vi "Pulse Accq -unphuck.vi"() -> ()   [LabVIEW 2009]
uses:
  5122-States.ctl
  <vilib>/Utility/file.llb/Write To Spreadsheet File (DBL).vi
  <instrlib>/niScope/Configure/Trigger/niScope Configure Trigger Edge.vi
  <instrlib>/niScope/Acquire/Fetch/niScope Multi Fetch WDT.vi
  <instrlib>/niScope/Controls/niScope vertical coupling.ctl
panel:
  out "wfm info":T1(array[cluster]) {"reserved2" format="%.2f"; "reserved1" format="%.2f"; "offset" format="%^.3e"; "gain" format="%^.3e"; "xIncrement" format="%^.3e"; "relativeInitialX" format="%^.3e"; "absoluteInitialX" format="%^.3e"}
  out "# Acquired":i32=100 caption="Number of Records Acquired"
  out "# Fetched":i32=100 caption="Number of Records Fetched"
  out "Last Record Fetched":waveform(dbl)[](graph)
  in  "Plot Data?":bool=TRUE
  out "error out":errorcluster {"code" format="%.0x"}
  out "sample mode":i32
  out "Acquisition Sequence":dbl[][](graph)
  out "Total Acquired Time":dbl[unit]
  out "Total Number of Datapoints":i32=1000000
  out "Total Experiment Time":dbl[unit]
  in  "Number of Pulses to Record":i32=1 caption="Number of Runs" format="%.0p"
  out "Raman Measurement File Root":path
  out "Phase-Frequency Pairs":path
  out "Shot Noise File":path
  out "Reference Pulse File":path
  out "Quadrature Pulses File":path
  out "Raw Phase, Trigger, Extracted Phase Data":path
  out "Data Directory":path
  out "Writing Phase to File":bool
  in  "Master Stop":bool
  in  "Memory Repetition Period":dbl[unit]=0.025
  out "Actual Sample Rate":dbl[unit]
  in  "Get Reference Parameters":bool
  out "Reference Pulse":dbl[](array[numeric])
  in  "Capture":bool
  out "Acquisitions Remaining":i32 caption="Number of Runs"
  out "Number of Samples per Pulse":i32
  in  "Vertical range (0 to 10V)":dbl[unit]=4.0 caption="Vertical Range (V)" format="%.2f"
  in  "Desired Sample Rate":dbl[unit]=100000000.0 caption="Min. Sample Rate" step=1.0 format="%.2p"
  in  "Vertical coupling":T2=1 caption="Vertical Coupling" items=["AC", "DC", "Ground"]
  in  "Acquisition Delay":dbl[unit] format="%.2f"
  in  "Channel":u16(ring) items=["0", "1"]
  out "Channel String":string
  in  "Acquisition Time per Pulse":dbl[unit]=0.0005 format="%#.2g"
  in  "Acquire Data":bool
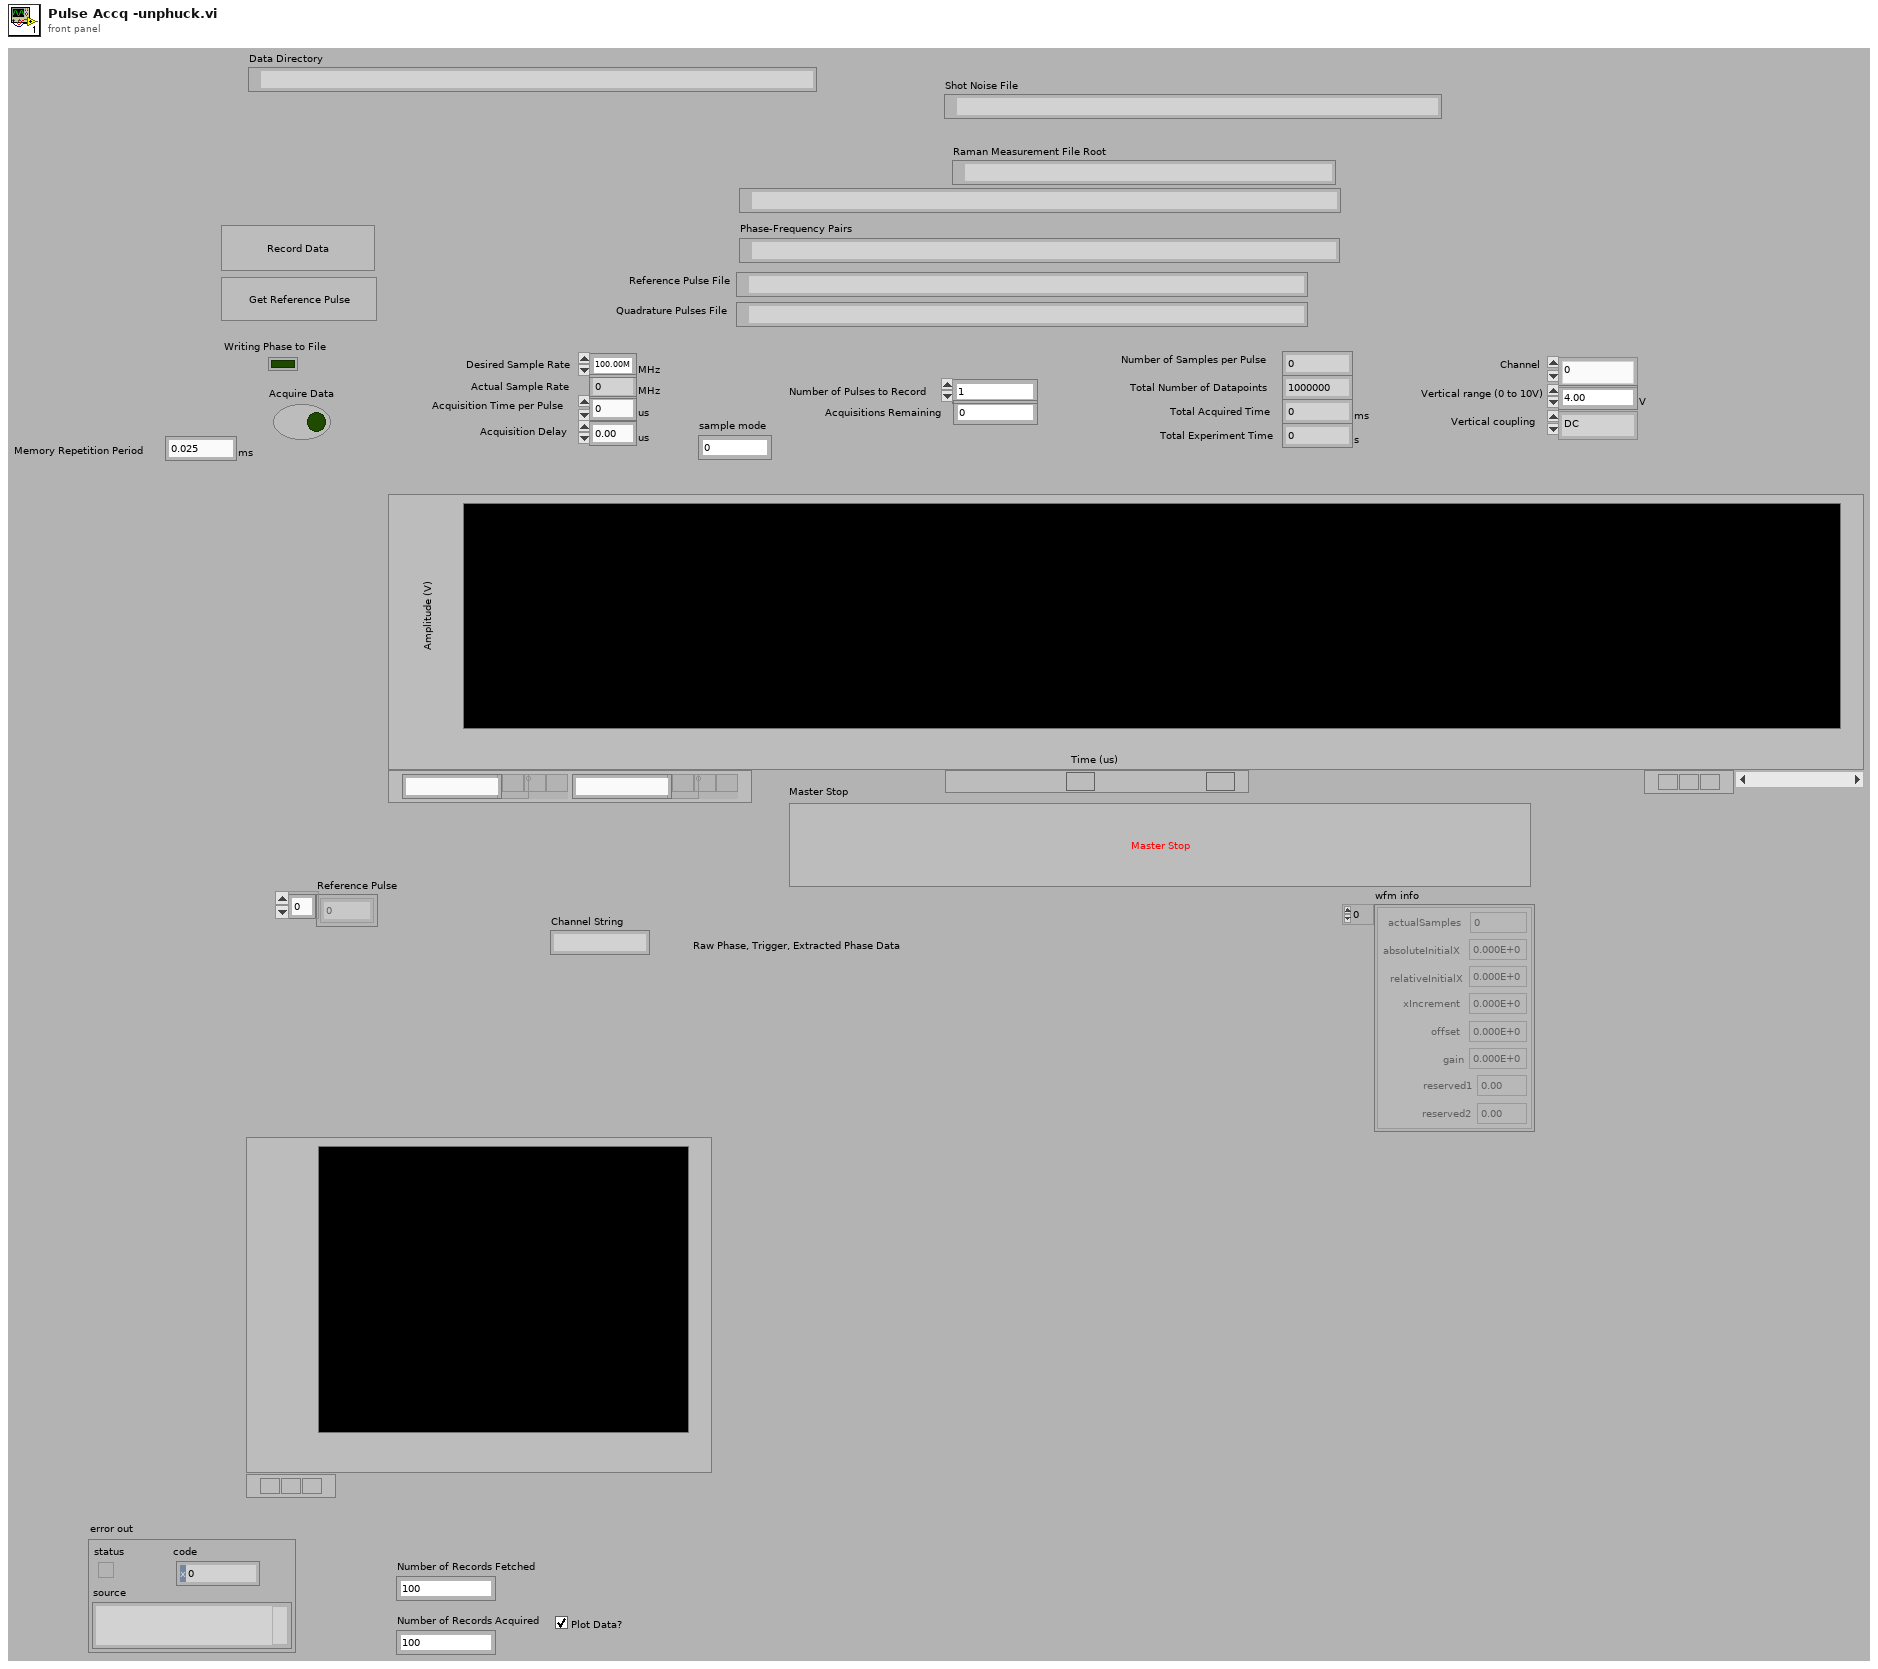
[diagram p1: front panel]
types:
  T1 = cluster{"actualSamples":i32, "absoluteInitialX":dbl, "relativeInitialX":dbl, "xIncrement":dbl, "offset":dbl, "gain":dbl, "reserved1":dbl, "reserved2":dbl}[]
  T2 = typedef "niScope vertical coupling.ctl" = i32
  T3 = enum16{"open", "open or create", "create or replace", "create", "open (read-only)"}
  T4 = enum16{"open", "replace", "create", "open or create", "replace or create", "replace or create with confirmation"}
  T5 = typedef "5122-States.ctl" = enum16{"Initialize Card", "Continuous Mode", "Fetch", "Snapshot Acquistion", "Standby", "Record DataFile", "Exit"}
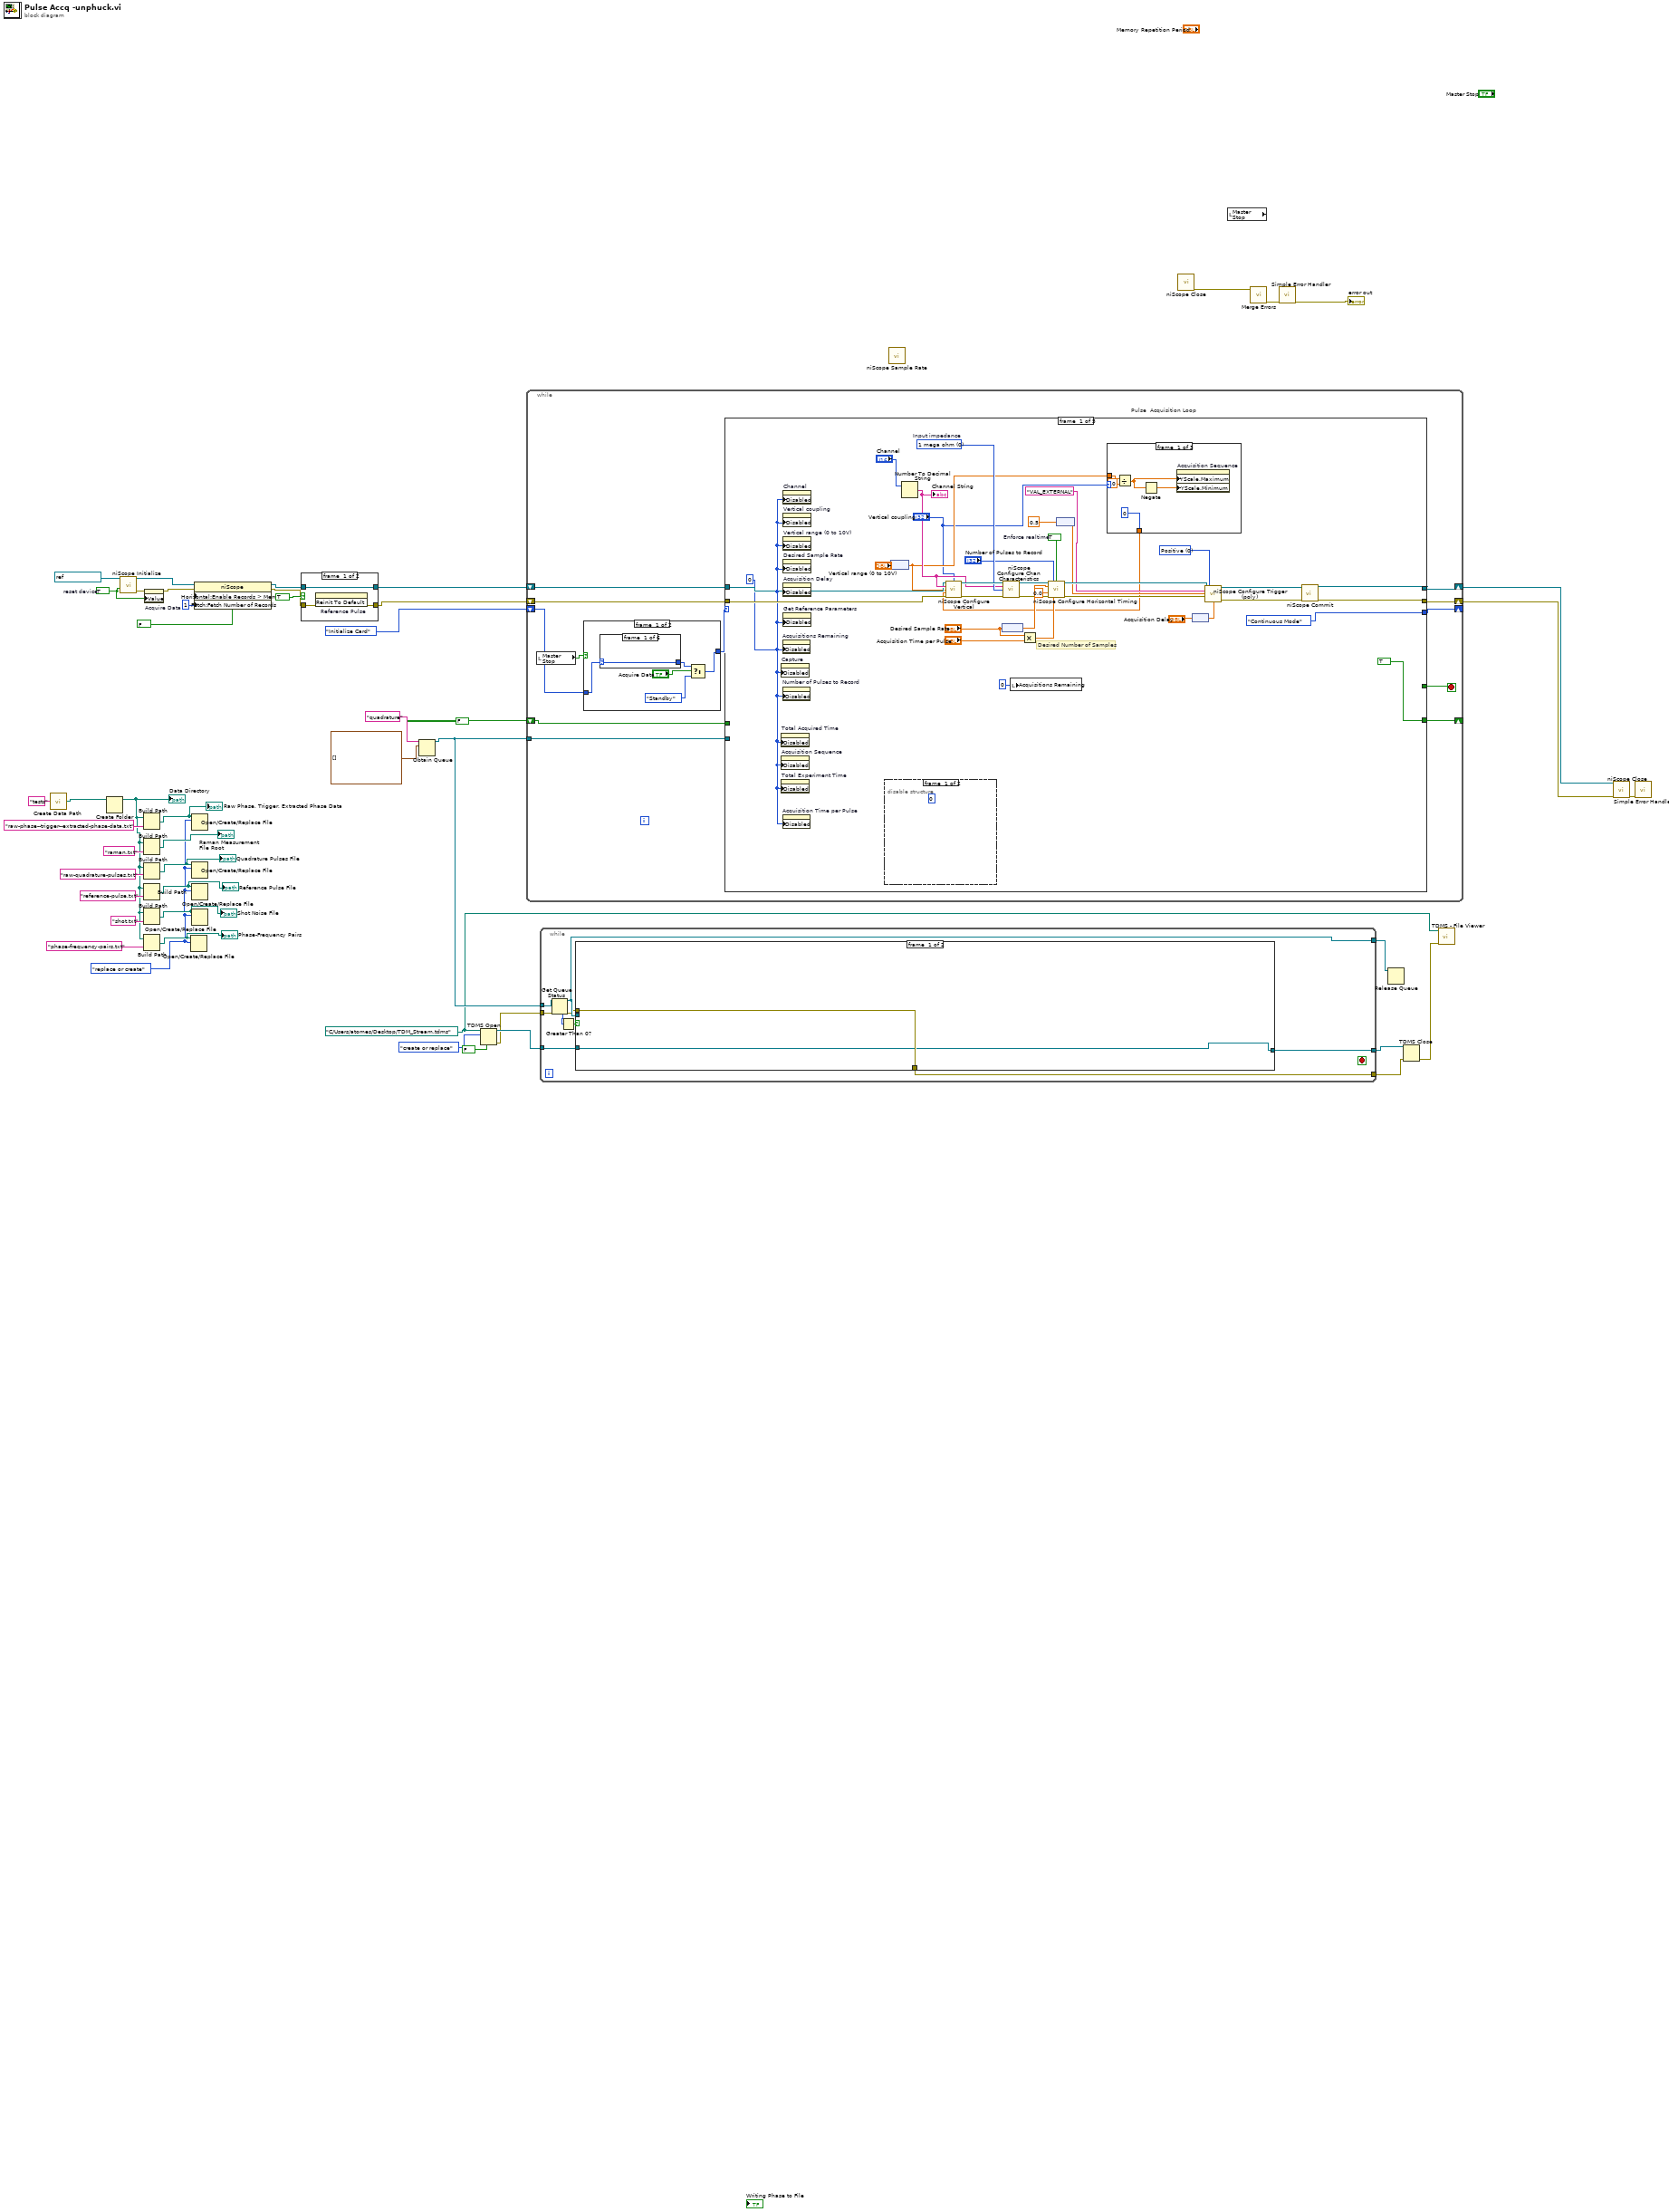
[diagram p0: block diagram]
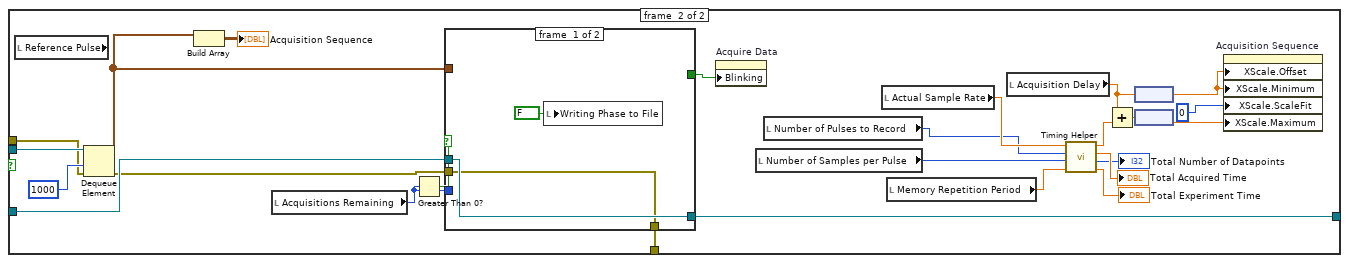
[diagram p2: hidden frame]
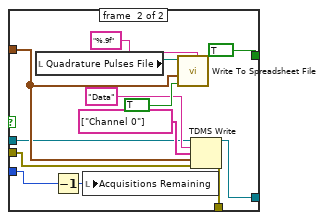
[diagram p3: hidden frame]
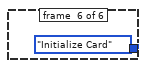
[diagram p9: hidden frame]
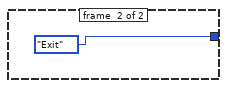
[diagram p10: hidden frame]
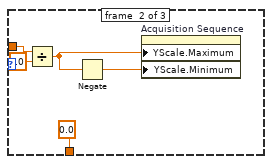
[diagram p12: hidden frame]
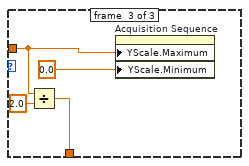
[diagram p13: hidden frame]
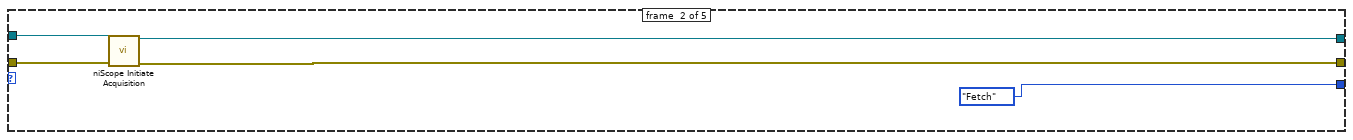
[diagram p14: hidden frame]
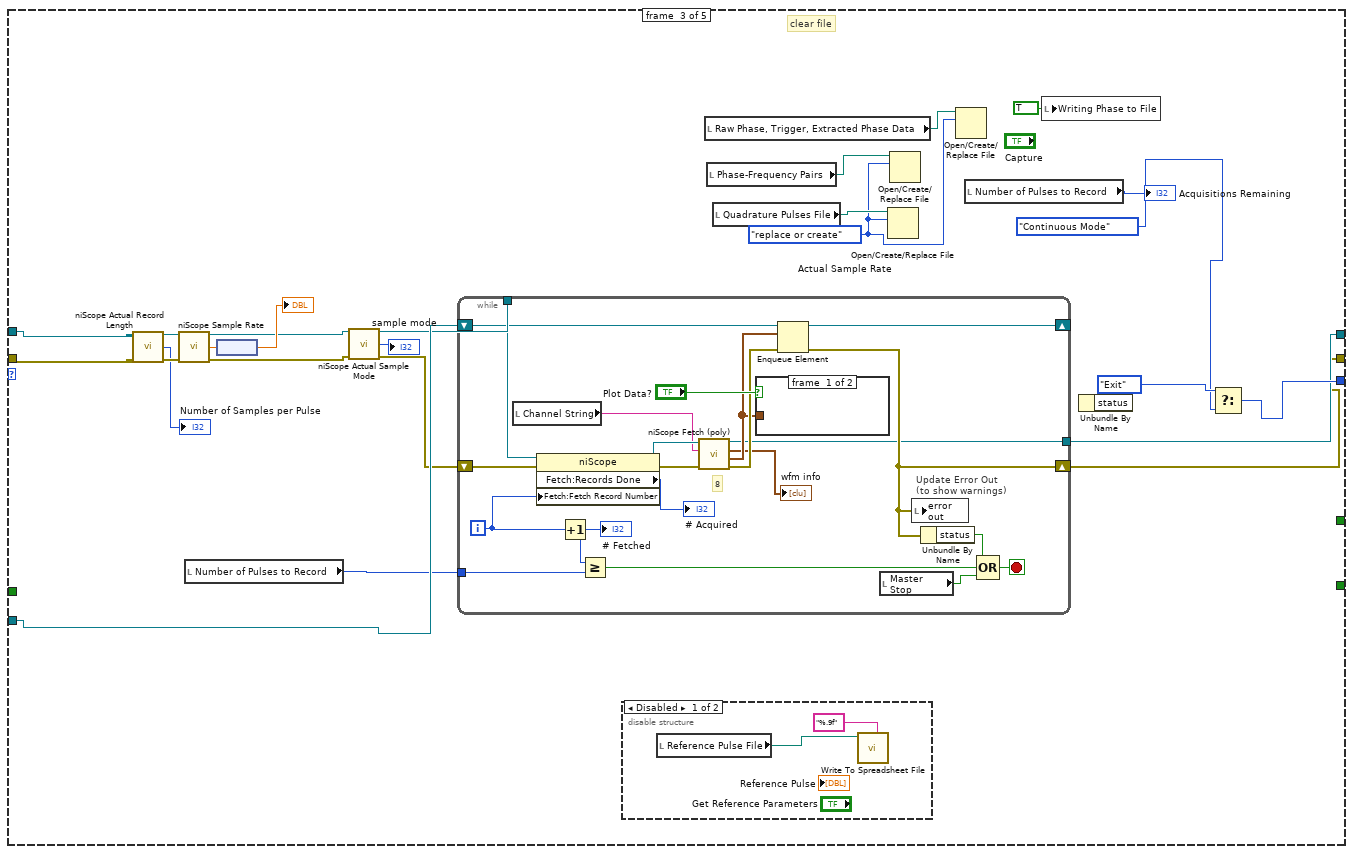
[diagram p15: hidden frame]
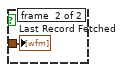
[diagram p17: hidden frame]
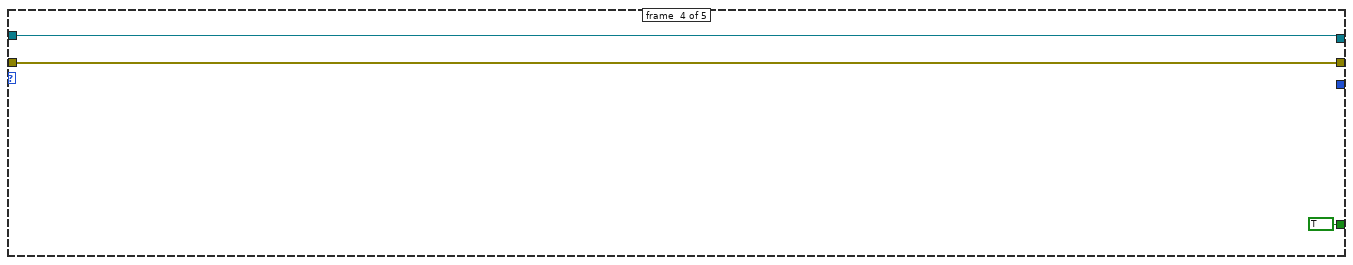
[diagram p18: hidden frame]
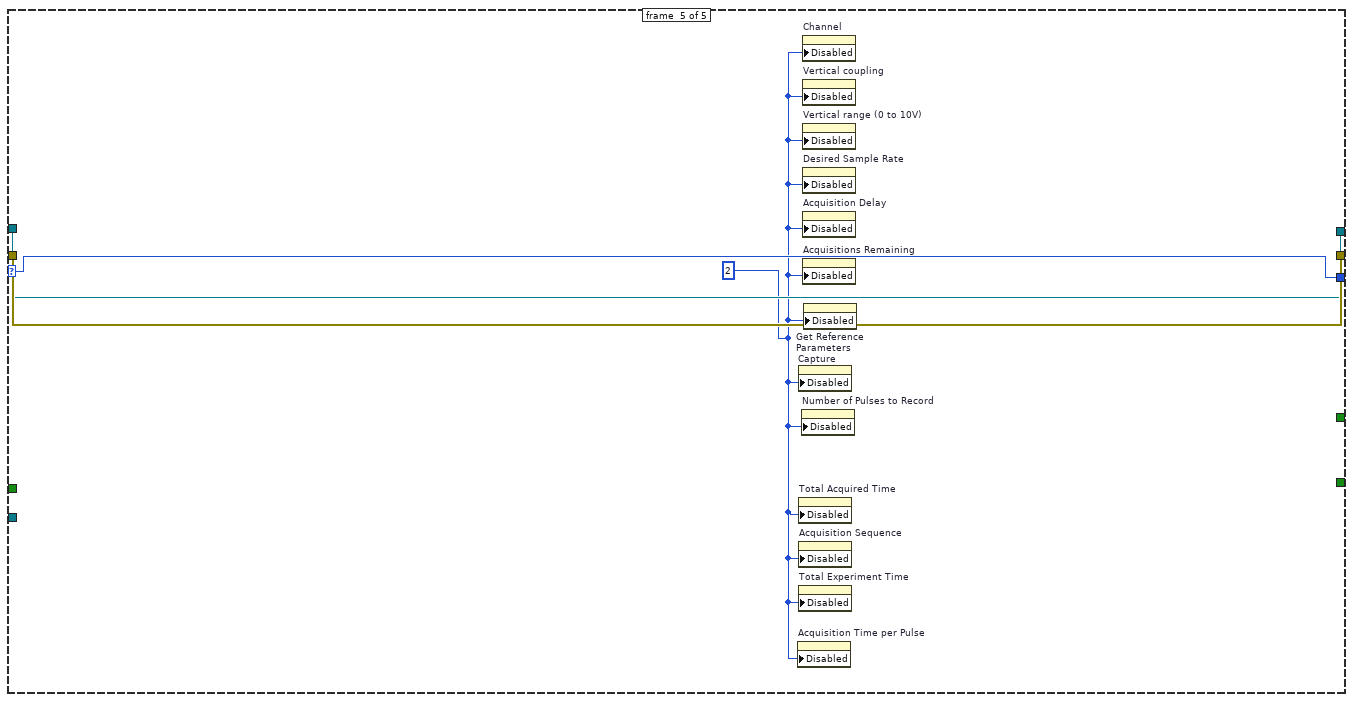
[diagram p19: hidden frame]
diagram:
  w4 = path "C:/Users/atomes/Desktop/TDM_Stream.tdms" ("selected path")
  w25 = T4."replace or create" ("operation (0:open)")
  w46 = TRUE  # reset device
  n1 = call "Create Data Path.vi"("Data Directory Name"="tests") -> ("appended path"=w36:path)
  n2 = Create Folder(path (use dialog)=w36) -> (created path=w27:path)  [unwired: 2 in, 2 out]
  "Data Directory" <- w27
  n3 = call <instrlib>:"niScope Initialize.vi"("resource name"=refnum<k15> "Acquisition" ("Resource name 5"), "reset device"=w46) -> ("instrument handle"=w17:refnum<k15>, "error out"=w47:errorcluster)  [unwired: 2 in, 10 out]
  n4 = Build Path(base path=w27, name or relative path="raw-phase--trigger--extracted-phase-data.txt") -> (appended path=w34:path)
  "Raw Phase, Trigger, Extracted Phase Data" <- w34
  n5 = Build Path(base path=w27, name or relative path="raman.txt") -> (appended path=→"Raman Measurement File Root":path)
  n6 = Build Path(base path=w27, name or relative path="raw-quadrature-pulses.txt") -> (appended path=w32:path)
  "Quadrature Pulses File" <- w32
  n7 = Build Path(base path=w27, name or relative path="reference-pulse.txt") -> (appended path=w31:path)
  "Reference Pulse File" <- w31
  n8 = Build Path(base path=w27, name or relative path="shot.txt") -> (appended path=w30:path)
  "Shot Noise File" <- w30
  n9 = Build Path(base path=w27, name or relative path="phase-frequency-pairs.txt") -> (appended path=w26:path)
  "Phase-Frequency Pairs" <- w26
  n10 = property on="Acquire Data" class="Bool (strict)"(error in=w47, "Value"=w46) -> (error out=w14:errorcluster)  [unwired: 1 in, 1 out]
  n11 = Open/Create/Replace File(file path (use dialog)=w26, operation (0:open)=w25) -> ()  [unwired: 4 in, 3 out]
  n12 = Open/Create/Replace File(file path (use dialog)=w34, operation (0:open)=w25) -> ()  [unwired: 4 in, 3 out]
  n13 = Open/Create/Replace File(file path (use dialog)=w32, operation (0:open)=w25) -> ()  [unwired: 4 in, 3 out]
  n14 = Open/Create/Replace File(file path (use dialog)=w31, operation (0:open)=w25) -> ()  [unwired: 4 in, 3 out]
  n15 = Open/Create/Replace File(file path (use dialog)=w30, operation (0:open)=w25) -> ()  [unwired: 4 in, 3 out]
  n16 = property class="niScope"(reference=w17, error in=w14, "Horizontal:Enable Records > Memory"=FALSE, "Fetch:Fetch Number of Records"=1) -> (reference out=w16:refnum<k15>, error out=w15:errorcluster)
  n17 = case shown="True" TRUE {
    tunnel: [w50 w52] -> w43
    tunnel: w16 -> [w50 w52]
    tunnel: [w49 w51] -> w42
    tunnel: w15 -> [w49 w51]
    frame #0 {
      n18 = invoke on="Reference Pulse" class="Arr (strict)" method="Reinit To Default"() -> ()  [unwired: 3 in, 3 out]
    }
    frame #1 {
    }
  }
  n19 = Obtain Queue(name (unnamed)="quadrature", element data type=waveform(dbl)[] [] ("wfm")) -> (queue out=w23:refnum<queue>)  [unwired: 3 in, 2 out]
  n20 = TDMS Open(6:FALSE ("disable buffering (T)"), 10:T3."create or replace" ("operation"), 11:w4) -> (0:w7:errorcluster, 3:w10:refnum<k34>)  [unwired: 3 in]
  n21 = while {
    shift-right: [w59] -> _
    shift-left: 5122-States."Initialize Card" ("Enum") -> [w57]
    shift-right: [w64] -> w21
    shift-left: w43 -> [w62]
    shift-right: [w63] -> w22
    shift-left: w42 -> [w61]
    shift-right: [w56] -> _
    shift-left: FALSE -> [w55]
    tunnel: w23 -> [w53]
    stop <- w60 stop-if-true
    # "Pulse  Acquisition Loop"
    n22 = local read "Master Stop"() -> (w54:bool)
    n23 = case shown="False" w54 {
      tunnel: [w66 5122-States."Exit" ("Enum")] -> w58
      tunnel: w57 -> [w69 _]
      frame #0 {
        n24 = case shown="\"Continuous Mode\"" w69 {
          selector: w69 -> [w70 w71 w72 w73 w74 _]
          tunnel: [w70 w71 w72 w73 w74 5122-States."Initialize Card" ("Enum")] -> w68
          frame #0 {
          }
          frame #1 {
          }
          frame #2 {
          }
          frame #3 {
          }
          frame #4 {
          }
          frame #5 {
          }
        }
        n25 = Select(t=w68, s="Acquire Data", f=5122-States."Standby" ("Enum")) -> (s? t:f=w66:T5)
      }
      frame #1 {
      }
    }
    n26 = case shown="\"Fetch\"" w58 {
      selector: w58 -> [_ _ _ _ w186]
      tunnel: [w94 w129 w140 w184 w187] -> w64
      tunnel: [w93 w130 w139 w183 w188] -> w63
      tunnel: w62 -> [w96 w132 w146 w184 w187]
      tunnel: w61 -> [w95 w131 w145 w183 w188]
      tunnel: [5122-States."Continuous Mode" ("Enum") 5122-States."Fetch" ("Enum") w157 _ w186] -> w59
      tunnel: [_ _ _ TRUE ("Acquire Data") _] -> w60
      tunnel: [TRUE _ _ _ _] -> w56
      tunnel: w55 -> [_ _ _ _ _]
      tunnel: w53 -> [_ _ w144 _ _]
      frame #0 {
        w80 = u8 0 ("Disabled")
        w104 = 0 items=["Positive", "Negative"] ("Trigger slope 6")
        w111 = TRUE  # Enforce realtime
        w107 = u32 0 items=["1 mega ohm", "75 ohms", "50 ohms"]  # Input impedance
        # "Desired Number of Samples"
        n27 = property on="Capture" class="Bool"("Disabled"=w80) -> ()  [unwired: 2 in, 2 out]
        n28 = property on="Total Acquired Time" class="DigNum (strict)"("Disabled"=w80) -> ()  [unwired: 2 in, 2 out]
        n29 = property on="Acquisition Sequence" class="WFGraph (strict)"("Disabled"=w80) -> ()  [unwired: 2 in, 2 out]
        n30 = property on="Total Experiment Time" class="DigNum (strict)"("Disabled"=w80) -> ()  [unwired: 2 in, 2 out]
        n31 = property on="Acquisitions Remaining" class="DigNum (strict)"("Disabled"=w80) -> ()  [unwired: 2 in, 2 out]
        n32 = property on="Number of Pulses to Record" class="DigNum (strict)"("Disabled"=w80) -> ()  [unwired: 2 in, 2 out]
        n33 = property on="Acquisition Time per Pulse" class="DigNum (strict)"("Disabled"=w80) -> ()  [unwired: 2 in, 2 out]
        n34 = property on="Channel" class="Ring (strict)"("Disabled"=w80) -> ()  [unwired: 2 in, 2 out]
        n35 = property on="Vertical coupling" class="Ring (strict)"("Disabled"=w80) -> ()  [unwired: 2 in, 2 out]
        n36 = property on="Vertical range (0 to 10V)" class="DigNum (strict)"("Disabled"=w80) -> ()  [unwired: 2 in, 2 out]
        n37 = property on="Desired Sample Rate" class="DigNum (strict)"("Disabled"=w80) -> ()  [unwired: 2 in, 2 out]
        n38 = property on="Acquisition Delay" class="DigNum (strict)"("Disabled"=w80) -> ()  [unwired: 2 in, 2 out]
        n39 = property on="Get Reference Parameters" class="Bool"("Disabled"=w80) -> ()  [unwired: 2 in, 2 out]
        n40 = disable-structure shown="Enabled" {
          frame #0 {
            w113 = 0
          }
          frame #1 {
          }
        }
        n41 = node("Vertical range (0 to 10V)") -> (w86:dbl)
        n42 = Number To Decimal String(number="Channel") -> (decimal integer string=w97:string)  [unwired: 1 out]
        "Channel String" <- w97
        n43 = node("Desired Sample Rate") -> (w91:dbl)
        n44 = local write "Acquisitions Remaining"(0 ("Acquisitions Remaining")) -> ()
        n45 = Multiply(x="Desired Sample Rate", y="Acquisition Time per Pulse") -> (x*y=w87:dbl)
        n46 = node(dbl[unit] 0.5 ("Trigger level")) -> (w99:dbl)
        n47 = case shown="1" "Vertical coupling" {
          tunnel: w86 -> [w118 w123 w126]
          tunnel: [0 0.0 w124] -> w83
          frame #0 {
            n48 = Divide(x=w118, y=2.0) -> (x/y=w116:dbl)
            n49 = Negate(x=w116) -> (-x=w115:dbl)
            n50 = property on="Acquisition Sequence" class="WFGraph (strict)"("YScale.Maximum"=w116, "YScale.Minimum"=w115) -> ()  [unwired: 2 in, 2 out]
          }
          frame #1 {
            n51 = Divide(x=w123, y=2.0) -> (x/y=w121:dbl)
            n52 = Negate(x=w121) -> (-x=w120:dbl)
            n53 = property on="Acquisition Sequence" class="WFGraph (strict)"("YScale.Maximum"=w121, "YScale.Minimum"=w120) -> ()  [unwired: 2 in, 2 out]
          }
          frame #2 {
            n54 = Divide(x=w126, y=2.0) -> (x/y=w124:dbl)
            n55 = property on="Acquisition Sequence" class="WFGraph (strict)"("YScale.Maximum"=w126, "YScale.Minimum"=0.0 ("Y Scale.Range:Minimum")) -> ()  [unwired: 2 in, 2 out]
          }
        }
        n56 = call <instrlib>:"niScope Configure Vertical.vi"("instrument handle"=w96, "vertical coupling"="Vertical coupling", "channels"=w97, "vertical range"=w86, "vertical offset"=w83, "error in"=w95) -> ("instrument handle out"=w110:refnum<k15>, "error out"=w109:errorcluster)  [unwired: 2 in, 6 out]
        n57 = call <instrlib>:"niScope Configure Chan Characteristics.vi"("instrument handle"=w110, "channels"=w97, "input impedance"=w107, "error in"=w109) -> ("instrument handle out"=w102:refnum<k15>, "error out"=w108:errorcluster)  [unwired: 1 in, 9 out]
        n58 = call <instrlib>:"niScope Configure Horizontal Timing.vi"("instrument handle"=w102, "number of records"="Number of Pulses to Record", "enforce realtime"=w111, "min sample rate"=w91, "reference position"=0.0, "error in"=w108, "min record length"=w87) -> ("instrument handle out"=w105:refnum<k15>, "error out"=w106:errorcluster)  [unwired: 7 out]
        n59 = node("Acquisition Delay") -> (w92:dbl)
        n60 = call-poly <instrlib>:"niScope Configure Trigger (poly).vi"("instrument handle"=w105, "trigger slope"=w104, "trigger source"="VAL_EXTERNAL" ("Trigger source"), "trigger level"=w99, "error in"=w106, "trigger delay"=w92) -> ("instrument handle out"=w79:refnum<k15>, "error out"=w78:errorcluster)  [unwired: 2 in, 6 out]
        n61 = call <instrlib>:"niScope Commit.vi"("instrument handle"=w79, "error in"=w78) -> ("instrument handle out"=w94:refnum<k15>, "error out"=w93:errorcluster)  [unwired: 12 out]
      }
      frame #1 {
        n62 = call <instrlib>:"niScope Initiate Acquisition.vi"("instrument handle"=w132, "error in"=w131) -> ("instrument handle out"=w129:refnum<k15>, "error out"=w130:errorcluster)  [unwired: 12 out]
      }
      frame #2 {
        w135 = T4."replace or create" ("operation (0:open)")
        # "clear file"
        n63 = call <instrlib>:"niScope Actual Record Length.vi"("instrument handle"=w146, "error in"=w145) -> ("instrument handle out"=w156:refnum<k15>, "actual record length"=→"Number of Samples per Pulse":i32, "error out"=w154:errorcluster)  [unwired: 11 out]
        n64 = call <instrlib>:"niScope Sample Rate.vi"("instrument handle"=w156, "error in"=w154) -> ("instrument handle out"=w149:refnum<k15>, "actual sample rate"=w153:dbl, "error out"=w148:errorcluster)  [unwired: 11 out]
        n65 = local read "Number of Pulses to Record"() -> (w143:i32)
        n66 = node(w153) -> (→"Actual Sample Rate":dbl[unit])
        n67 = call <instrlib>:"niScope Actual Sample Mode.vi"("instrument handle"=w149, "error in"=w148) -> ("instrument handle out"=w142:refnum<k15>, "sample mode"=→"sample mode":i32, "error out"=w141:errorcluster)  [unwired: 11 in]
        n68 = while {
          tunnel: w143 -> [w180]
          tunnel: [w164] -> w140
          shift-right: [w167] -> _
          shift-left: w144 -> [w170]
          shift-right: [w168] -> w139
          shift-left: w141 -> [w171]
          tunnel: w142 -> [w160]
          i -> [w175]
          stop <- w179 stop-if-true
          # "8"
          # "Update Error Out\n(to show warnings)"
          n69 = local read "Channel String"() -> (w162:string)
          n70 = property class="niScope"(reference=w160, error in=w171, "Fetch:Fetch Record Number"=w175) -> (reference out=w172:refnum<k15>, error out=w174:errorcluster, "Fetch:Records Done"=→"# Acquired":i32)
          n71 = Increment(x=w175) -> (x+1=w177:i32)
          "# Fetched" <- w177
          n72 = Greater Or Equal?(x=w177, y=w180) -> (x >= y?=w165:bool)
          n73 = call-poly <instrlib>:"niScope Fetch (poly).vi"("error in"=w174, "channels"=w162, "instrument handle"=w172) -> ("error out"=w169:errorcluster, "wfm"=w166:waveform(dbl)[], "wfm info"=→"wfm info":T1, "instrument handle out"=w164:refnum<k15>)  [unwired: 3 in, 2 out]
          n74 = case shown="True" "Plot Data?" {
            tunnel: w166 -> [_ w181]
            frame #0 {
            }
            frame #1 {
              "Last Record Fetched" <- w181
            }
          }
          n75 = Enqueue Element(queue=w170, element=w166, error in (no error)=w169) -> (queue out=w167:refnum<queue>, error out=w168:errorcluster)  [unwired: 2 out]
          n76 = local read "Master Stop"() -> (w163:bool)
          n77 = local write "error out"(w168) -> ()
          n78 = Unbundle By Name(w168) -> ("status"=w173:bool)
          n79 = Compound Arithmetic op=OR(w173, w165, w163) -> (w179:bool)
        }
        n80 = disable-structure shown="Disabled" {
          frame #0 {
            n81 = local read "Reference Pulse File"() -> (w159:path)
            n82 = call-poly <vilib>:"Write To Spreadsheet File.vi"("format (%.3f)"="%.9f", "file path (dialog if empty)"=w159) -> ()  [unwired: 4 in, 3 out]
          }
          frame #1 {
          }
        }
        n83 = local read "Raw Phase, Trigger, Extracted Phase Data"() -> (w134:path)
        n84 = local read "Phase-Frequency Pairs"() -> (w133:path)
        n85 = local read "Quadrature Pulses File"() -> (w136:path)
        n86 = Open/Create/Replace File(file path (use dialog)=w136, operation (0:open)=w135) -> ()  [unwired: 4 in, 3 out]
        n87 = Open/Create/Replace File(file path (use dialog)=w133, operation (0:open)=w135) -> ()  [unwired: 4 in, 3 out]
        n88 = Open/Create/Replace File(file path (use dialog)=w134, operation (0:open)=w135) -> ()  [unwired: 4 in, 3 out]
        n89 = local read "Number of Pulses to Record"() -> (→"Acquisitions Remaining":i32)
        n90 = local write "Writing Phase to File"(TRUE ("Write Phase to File")) -> ()
        n91 = Unbundle By Name() -> ()  [unwired: 1 in, 1 out]
        n92 = Select(t=5122-States."Exit" ("Enum"), f=5122-States."Continuous Mode" ("Enum")) -> (s? t:f=w157:T5)  [unwired: 1 in]
      }
      frame #3 {
      }
      frame #4 {
        w185 = u8 2 ("Disabled")
        n93 = property on="Acquisition Time per Pulse" class="DigNum (strict)"("Disabled"=w185) -> ()  [unwired: 2 in, 2 out]
        n94 = property on="Capture" class="Bool"("Disabled"=w185) -> ()  [unwired: 2 in, 2 out]
        n95 = property on="Total Acquired Time" class="DigNum (strict)"("Disabled"=w185) -> ()  [unwired: 2 in, 2 out]
        n96 = property on="Acquisition Sequence" class="WFGraph (strict)"("Disabled"=w185) -> ()  [unwired: 2 in, 2 out]
        n97 = property on="Total Experiment Time" class="DigNum (strict)"("Disabled"=w185) -> ()  [unwired: 2 in, 2 out]
        n98 = property on="Number of Pulses to Record" class="DigNum (strict)"("Disabled"=w185) -> ()  [unwired: 2 in, 2 out]
        n99 = property on="Channel" class="Ring (strict)"("Disabled"=w185) -> ()  [unwired: 2 in, 2 out]
        n100 = property on="Vertical coupling" class="Ring (strict)"("Disabled"=w185) -> ()  [unwired: 2 in, 2 out]
        n101 = property on="Vertical range (0 to 10V)" class="DigNum (strict)"("Disabled"=w185) -> ()  [unwired: 2 in, 2 out]
        n102 = property on="Desired Sample Rate" class="DigNum (strict)"("Disabled"=w185) -> ()  [unwired: 2 in, 2 out]
        n103 = property on="Acquisition Delay" class="DigNum (strict)"("Disabled"=w185) -> ()  [unwired: 2 in, 2 out]
        n104 = property on="Acquisitions Remaining" class="DigNum (strict)"("Disabled"=w185) -> ()  [unwired: 2 in, 2 out]
        n105 = property on="Get Reference Parameters" class="Bool"("Disabled"=w185) -> ()  [unwired: 2 in, 2 out]
      }
    }
  }
  n106 = while {
    tunnel: w23 -> [w197]
    tunnel: w10 -> [w194]
    tunnel: [w193] -> w9
    tunnel: [w192] -> w8
    tunnel: w7 -> [w191]
    tunnel: [w189] -> w6
    stop <- _ stop-if-true
    n107 = Get Queue Status(queue=w197, error in (no error)=w191) -> (queue out=w192:refnum<queue>, error out=w190:errorcluster, # elements in queue=w196:i32)  [unwired: 6 out]
    n108 = Greater Than 0?(x=w196) -> (x > 0?=w195:bool)
    n109 = case shown="True" w195 {
      tunnel: w192 -> [_ w205]
      tunnel: w194 -> [w198 w204]
      tunnel: [w198 w203] -> w193
      tunnel: w190 -> [w199 w202]
      tunnel: [w199 w200] -> w189
      frame #0 {
      }
      frame #1 {
        n110 = local read "Reference Pulse"() -> ()  [unwired: 1 out]
        n111 = Dequeue Element(queue=w205, timeout in ms (-1)=1000, error in (no error)=w202) -> (element=w220:waveform(dbl)[], error out=w201:errorcluster)  [unwired: 2 out]
        n112 = Build Array(w220) -> (→"Acquisition Sequence":waveform(dbl)[][])  [unwired: 1 in]
        n113 = local read "Acquisitions Remaining"() -> (w223:i32)
        n114 = Greater Than 0?(x=w223) -> (x > 0?=w222:bool)
        n115 = case shown="True" w222 {
          tunnel: [_ TRUE ("Blinking")] -> w221
          tunnel: w223 -> [_ w238]
          tunnel: w220 -> [_ w232]
          tunnel: w204 -> [w226 w231]
          tunnel: [w226 w230] -> w203
          tunnel: w201 -> [w225 w229]
          tunnel: [w225 w228] -> w200
          frame #0 {
            n116 = local write "Writing Phase to File"(FALSE ("Save to File")) -> ()
          }
          frame #1 {
            n117 = local read "Quadrature Pulses File"() -> (w237:path)
            n118 = Decrement(x=w238) -> (x-1=w240:i32)
            n119 = local write "Acquisitions Remaining"(w240) -> ()
            n120 = call-poly <vilib>:"Write To Spreadsheet File.vi"("format (%.3f)"="%.9f", "append to file? (new file:F)"=TRUE, "1D data"=w232, "file path (dialog if empty)"=w237) -> ()  [unwired: 2 in, 3 out]
            n121 = TDMS Write(0:w231, 5:"Data" ("group name in"), 7:string[] ["Channel 0"] ("channel name(s) in (Untitled)"), 9:w232, 11:w229) -> (4:w230:refnum<k34>, 15:w228:errorcluster)  [unwired: 1 in, 2 out]
          }
        }
        n122 = property on="Acquire Data" class="Bool (strict)"("Blinking"=w221) -> ()  [unwired: 2 in, 2 out]
        n123 = local read "Number of Samples per Pulse"() -> (w219:i32)
        n124 = local read "Number of Pulses to Record"() -> (w206:i32)
        n125 = local read "Actual Sample Rate"() -> (w218:dbl[unit])
        n126 = local read "Memory Repetition Period"() -> (w208:dbl[unit])
        n127 = local read "Acquisition Delay"() -> (w212:dbl[unit])
        n128 = call "Timing Helper.vi"("Repetition Period"=w208, "Number of points per run"=w219, "Number of runs"=w206, "Sample rate"=w218) -> ("Total Experiment Time"=→"Total Experiment Time":dbl[unit], "Total Number of Datapoints"=→"Total Number of Datapoints":i32, "Total Acquired Time"=→"Total Acquired Time":dbl[unit], "Acquisition Time per Run"=w217:dbl[unit])
        n129 = Add(x=w212, y=w217) -> (x+y=w213:dbl[unit])
        n130 = node(w212) -> (w209:dbl)
        n131 = node(w213) -> (w210:dbl)
        n132 = property on="Acquisition Sequence" class="WFGraph (strict)"("XScale.Offset"=w209, "XScale.Minimum"=w209, "XScale.ScaleFit"=u8 0 ("X Scale.Scale Fit"), "XScale.Maximum"=w210) -> ()  [unwired: 2 in, 2 out]
      }
    }
  }
  n133 = call <instrlib>:"niScope Sample Rate.vi"() -> ()  [unwired: 2 in, 14 out]
  n134 = call <instrlib>:"niScope Close.vi"() -> ("error out"=w2:errorcluster)  [unwired: 2 in, 13 out]
  n135 = local read "Master Stop"() -> ()  [unwired: 1 out]
  n136 = call <vilib>:"Merge Errors.vi"("error in 1 (no error)"=w2) -> ("error out"=w3:errorcluster)  [unwired: 3 in, 3 out]
  n137 = call <vilib>:"Simple Error Handler.vi"("error in (no error)"=w3) -> ("error out"=→"error out":errorcluster)  [unwired: 1 in, 7 out]
  n138 = Release Queue(queue=w8) -> ()  [unwired: 1 in, 4 out]
  n139 = TDMS Close(8:w6, 11:w9) -> (0:w5:errorcluster)
  n140 = call <vilib>:"TDMS - File Viewer.vi"("error in (no error)"=w5, "file path"=w4) -> ()  [unwired: 6 out]
  n141 = call <instrlib>:"niScope Close.vi"("instrument handle"=w21, "error in"=w22) -> ("error out"=w20:errorcluster)  [unwired: 13 out]
  n142 = call <vilib>:"Simple Error Handler.vi"("error in (no error)"=w20) -> ()  [unwired: 1 in, 8 out]
